vi "Get All Data.vi"(0 "Arduino Resource":T3={"VISA resource"="", "Board Type"=enum."Uno", "Connection Type"=enum."USB / Serial", "Bytes Per Packet (15)"=15}, 5 "Device Address":T1=104 items=["0x68"=104, "0x69"=105], 11 "error in (no error)":errorcluster) -> (4 "Arduino Resource":T3={"VISA resource"="", "Board Type"=enum."Uno", "Connection Type"=enum."USB / Serial", "Bytes Per Packet (15)"=15}, 6 "Accel Data":T2, 8 "Temperature (°C)":dbl, 10 "Gyro Data":T2, 15 "error out":errorcluster)   [LabVIEW 2012, in "LIFA MPU-60X0.lvlib"]
uses:
  LIFA MPU-60X0.lvlib
  <vilib>/LabVIEW Interface for Arduino/Type Defs/Arduino Resource.ctl
  <vilib>/LabVIEW Interface for Arduino/Type Defs/Board Type.ctl
  DeviceAddresses.ctl
  RegisterAddresses.ctl
  <vilib>/LabVIEW Interface for Arduino/LabVIEW Interface for Arduino.lvlib
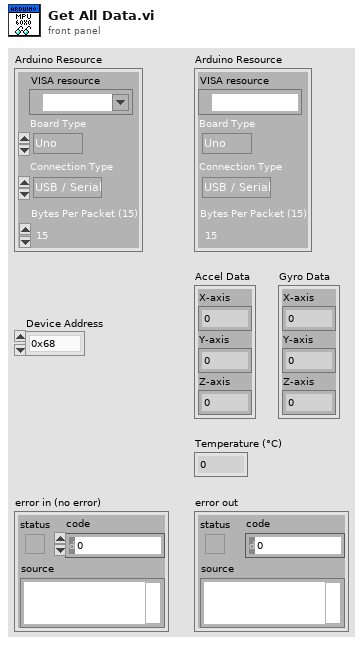
[diagram p1: front panel]
types:
  T1 = typedef "LIFA MPU-60X0.lvlib/DeviceAddresses.ctl" = u8
  T2 = cluster{"X-axis":i16, "Y-axis":i16, "Z-axis":i16}
  T3 = typedef "LabVIEW Interface for Arduino.lvlib/Arduino Resource.ctl" = cluster{"VISA resource":refnum<visa-resource-name>, "Board Type":T4, "Connection Type":enum8{"USB / Serial"}, "Bytes Per Packet (15)":u8}
  T4 = typedef "LabVIEW Interface for Arduino.lvlib/Board Type.ctl" = enum16{"Uno", "Dimuelanove w/Atmega 328", "Mega 2560"}
  T5 = typedef "LIFA MPU-60X0.lvlib/RegisterAddresses.ctl" = u16
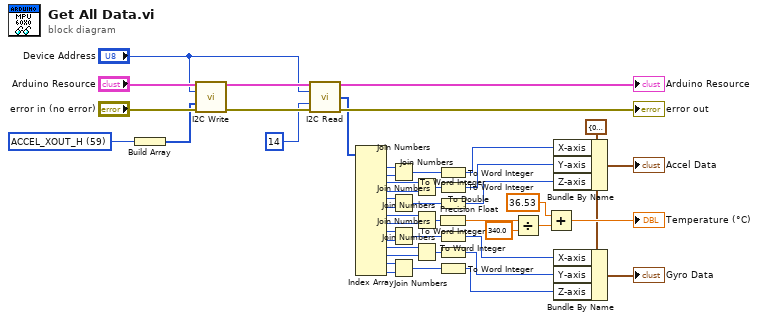
[diagram p0: block diagram]
diagram:
  w5 = T2 {"X-axis"=0, "Y-axis"=0, "Z-axis"=0} ("input cluster")
  w40 = T5 59 items=["SELF_TEST_X"=13, "SELF_TEST_Y"=14, "SELF_TEST_Z"=15, "SELF_TEST_A"=16, "SMPLRT_DIV"=25, "CONFIG"=26, "GYRO_CONFIG"=27, "ACCEL_CONFIG"=28, "MOT_THR"=31, "FIFO_EN"=35, "I2C_MST_CTRL"=36, "I2C_SLV0_ADDR"=37, "I2C_SLV0_REG"=38, "I2C_SLV0_CTRL"=39, "I2C_SLV1_ADDR"=40, "I2C_SLV1_REG"=41, "I2C_SLV1_CTRL"=42, "I2C_SLV2_ADDR"=43, "I2C_SLV2_REG"=44, "I2C_SLV2_CTRL"=45, "I2C_SLV3_ADDR"=46, "I2C_SLV3_REG"=47, "I2C_SLV3_CTRL"=48, "I2C_SLV4_ADDR"=49, "I2C_SLV4_REG"=50, "I2C_SLV4_DO"=51, "I2C_SLV4_CTRL"=52, "I2C_SLV4_DI"=53, "I2C_MST_STATUS"=54, "INT_PIN_CFG"=55, "INT_ENABLE"=56, "INT_STATUS"=58, "ACCEL_XOUT_H"=59, "ACCEL_XOUT_L"=60, "ACCEL_YOUT_H"=61, "ACCEL_YOUT_L"=62, "ACCEL_ZOUT_H"=63, "ACCEL_ZOUT_L"=64, "TEMP_OUT_H"=65, "TEMP_OUT_L"=66, "GYRO_XOUT_H"=67, "GYRO_XOUT_L"=68, "GYRO_YOUT_H"=69, "GYRO_YOUT_L"=70, "GYRO_ZOUT_H"=71, "GYRO_ZOUT_L"=72, "EXT_SENS_DATA_00"=73, "EXT_SENS_DATA_01"=74, "EXT_SENS_DATA_02"=75, "EXT_SENS_DATA_03"=76, "EXT_SENS_DATA_04"=77, "EXT_SENS_DATA_05"=78, "EXT_SENS_DATA_06"=79, "EXT_SENS_DATA_07"=80, "EXT_SENS_DATA_08"=81, "EXT_SENS_DATA_09"=82, "EXT_SENS_DATA_10"=83, "EXT_SENS_DATA_11"=84, "EXT_SENS_DATA_12"=85, "EXT_SENS_DATA_13"=86, "EXT_SENS_DATA_14"=87, "EXT_SENS_DATA_15"=88, "EXT_SENS_DATA_16"=89, "EXT_SENS_DATA_17"=90, "EXT_SENS_DATA_18"=91, "EXT_SENS_DATA_19"=92, "EXT_SENS_DATA_20"=93, "EXT_SENS_DATA_21"=94, "EXT_SENS_DATA_22"=95, "EXT_SENS_DATA_23"=96, "I2C_SLV0_DO"=99, "I2C_SLV1_DO"=100, "I2C_SLV2_DO"=101, "I2C_SLV3_DO"=102, "I2C_MST_DELAY_CTRL"=103, "SIGNAL_PATH_RESET"=104, "MOT_DETECT_CTRL"=105, "USER_CTRL"=106, "PWR_MGMT_1"=107, "PWR_MGMT_2"=108, "FIFO_COUNTH"=114, "FIFO_COUNTL"=115, "FIFO_R_W"=116, "WHO_AM_I"=117] ("Register Addresses")
  n1 = Build Array(w40) -> (w39:T5[])
  n2 = call <vilib>:"I2C Write.vi"("Arduino Resource"="Arduino Resource", "Address (0)"="Device Address", "I2C Data Bytes"=w39, "error in"="error in (no error)") -> ("Arduino Resource"=w46:T3, "error out"=w45:errorcluster)  [unwired: 10 in]
  n3 = call <vilib>:"I2C Read.vi"("Arduino Resource"=w46, "Address (0)"="Device Address", "Bytes To Read"=u8 14, "error in"=w45) -> ("Arduino Resource"=→"Arduino Resource":T3, "I2C Data"=w36:u8[], "error out"=→"error out":errorcluster)  [unwired: 9 in]
  n4 = Index Array(array=w36) -> (element #1=w35:u8, element #2=w34:u8, element #3=w33:u8, element #4=w32:u8, element #5=w31:u8, element #6=w30:u8, element #7=w29:u8, element #8=w28:u8, element #9=w27:u8, element #10=w26:u8, element #11=w25:u8, element #12=w24:u8, element #13=w23:u8, element #14=w22:u8)  [unwired: 14 in]
  n5 = Join Numbers(hi=w35, lo=w34) -> ((hi.lo)=w20:u16)
  n6 = Join Numbers(hi=w31, lo=w30) -> ((hi.lo)=w19:u16)
  n7 = Join Numbers(hi=w27, lo=w26) -> ((hi.lo)=w15:u16)
  n8 = Join Numbers(hi=w23, lo=w22) -> ((hi.lo)=w16:u16)
  n9 = Join Numbers(hi=w33, lo=w32) -> ((hi.lo)=w21:u16)
  n10 = Join Numbers(hi=w29, lo=w28) -> ((hi.lo)=w18:u16)
  n11 = Join Numbers(hi=w25, lo=w24) -> ((hi.lo)=w17:u16)
  n12 = To Word Integer(number=w20) -> (16bit integer=w9:i16)
  n13 = To Word Integer(number=w21) -> (16bit integer=w8:i16)
  n14 = To Word Integer(number=w19) -> (16bit integer=w7:i16)
  n15 = To Double Precision Float(number=w18) -> (double precision float=w14:dbl)
  n16 = To Word Integer(number=w15) -> (16bit integer=w4:i16)
  n17 = To Word Integer(number=w17) -> (16bit integer=w3:i16)
  n18 = To Word Integer(number=w16) -> (16bit integer=w2:i16)
  n19 = Divide(x=w14, y=340.0) -> (x/y=w12:dbl)
  n20 = Add(x=36.53, y=w12) -> (x+y=→"Temperature (°C)":dbl)
  n21 = Bundle By Name(cluster=w5, "X-axis"=w9, "Y-axis"=w8, "Z-axis"=w7) -> (→"Accel Data":T2)
  n22 = Bundle By Name(cluster=w5, "X-axis"=w4, "Y-axis"=w3, "Z-axis"=w2) -> (→"Gyro Data":T2)
